vi "Is VI Runnable.vi"(8 "error in (no error)":errorcluster, 11 "selected path":path) -> (0 "error out":errorcluster)   [LabVIEW 2014, in "Raspberry Pi Compatible Compiler for LabVIEW.lvlib"]
uses:
  Raspberry Pi Compatible Compiler for LabVIEW.lvlib
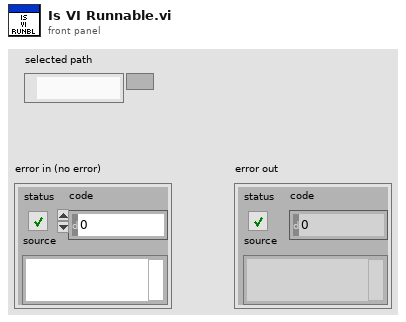
[diagram p1: front panel]
types:
  T1 = enum32{"Bad", "Idle", "Run top level", "Running"}
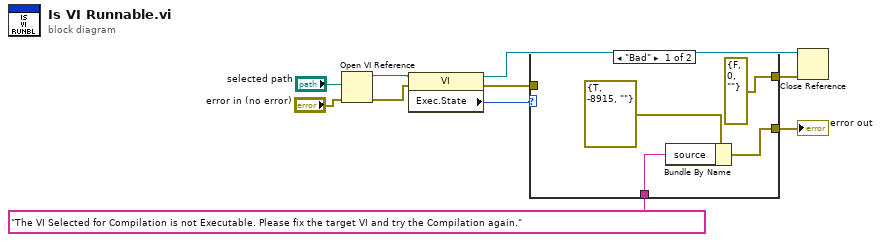
[diagram p0: block diagram]
diagram:
  n1 = Open VI Reference(vi path="selected path", error in (no error)="error in (no error)") -> (vi reference=w4:refnum<vi>, error out=w3:errorcluster)  [unwired: 4 in]
  n2 = property class="VI"(reference=w4, error in=w3) -> (reference out=w2:refnum<vi>, error out=w8:errorcluster, "Exec.State"=w9:T1)
  n3 = case shown="\"Bad\"" w9 {
    tunnel: [w13 w15] -> w6
    tunnel: w8 -> [_ w15]
    tunnel: "The VI Selected for Compilation is not Executable. Please fix the target VI and try the Compilation again." -> [w12 _]
    tunnel: [errorcluster {"status"=FALSE, "code"=0, "source"=""} ("error out") w15] -> w1
    frame "Bad" {
      n4 = Bundle By Name(cluster=errorcluster {"status"=TRUE, "code"=-8915, "source"=""} ("error in (no error)"), "source"=w12) -> (w13:errorcluster)
    }
    frame "Idle", Default {
    }
  }
  "error out" <- w6
  n5 = Close Reference(reference=w2, error in (no error)=w1) -> ()  [unwired: 1 out]
